vi "Config Dialog.vi"(8 "error in (no error)":errorcluster, 11 "DataGrid Config in":refnum<class "DataGrid Config.lvclass">) -> (0 "error out":errorcluster, 3 "DataGrid Config out":refnum<class "DataGrid Config.lvclass">)   [LabVIEW 2018, in "DataGrid Config Dialog.lvclass"]
uses:
  DataGrid Config Dialog.lvclass
  DataGrid Config/DataGrid Config.lvclass
  DataGrid Config Dialog.lvclass/DataGrid Config Dialog.ctl
panel:
  in  "Down":bool
  in  "Up":bool
  in  "Remove":bool
  in  "Add":bool
  in  "Selection":i32(listbox)
  in  "OK":bool
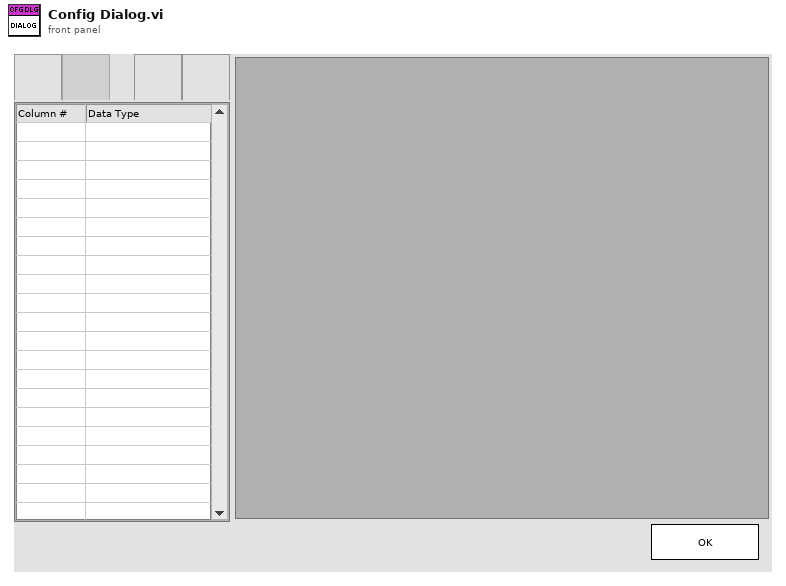
[diagram p1: front panel]
types:
  T1 = typedef "LVPoint32TypeDef.ctl" = cluster{"Horizontal":i32, "Vertical":i32}
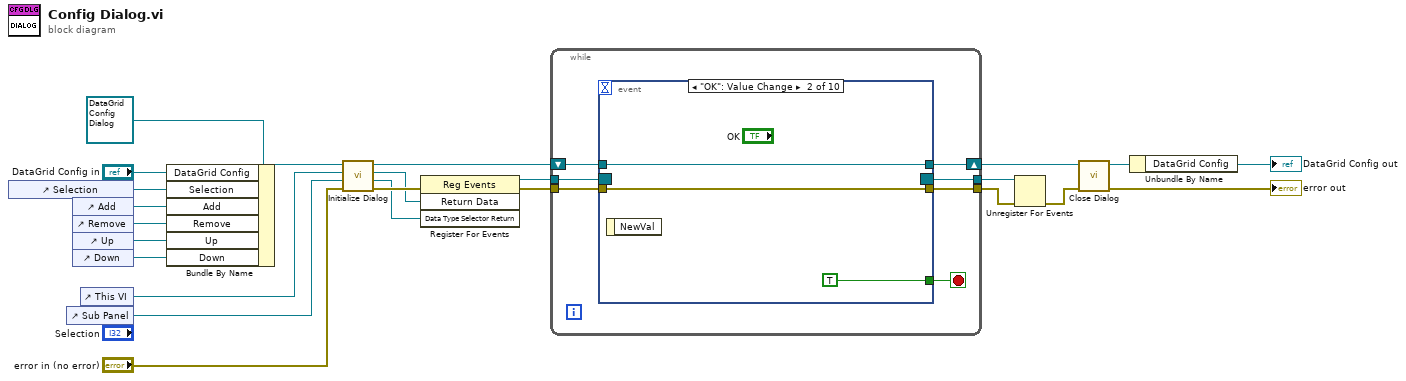
[diagram p0: block diagram]
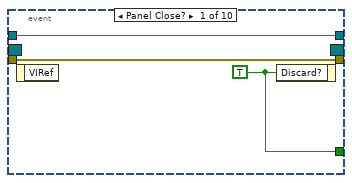
[diagram p2: hidden frame]
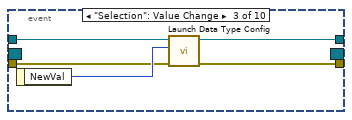
[diagram p3: hidden frame]
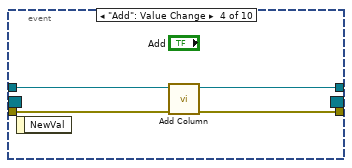
[diagram p4: hidden frame]
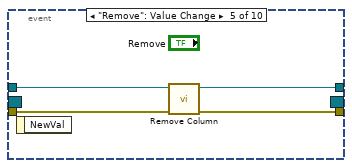
[diagram p5: hidden frame]
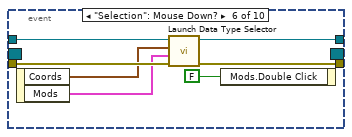
[diagram p6: hidden frame]
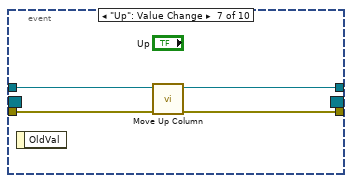
[diagram p7: hidden frame]
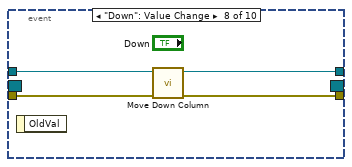
[diagram p8: hidden frame]
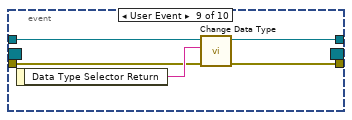
[diagram p9: hidden frame]
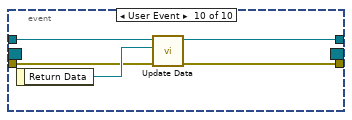
[diagram p10: hidden frame]
diagram:
  n1 = control-ref of="Selection"() -> (w22:refnum<vi>)
  n2 = control-ref of="Sub Panel"() -> (w21:refnum<vi>)
  n3 = control-ref of="Add"() -> (w11:refnum<vi>)
  n4 = control-ref of="Remove"() -> (w10:refnum<vi>)
  n5 = control-ref of="Up"() -> (w7:refnum<vi>)
  n6 = control-ref of="Down"() -> (w6:refnum<vi>)
  n7 = control-ref of="This VI"() -> (w20:refnum<vi>)
  n8 = Bundle By Name(cluster=refnum<class "DataGrid Config Dialog.lvclass"> refnum ("DataGrid Config Dialog.lvclass"), "DataGrid Config"="DataGrid Config in", "Selection"=w22, "Add"=w11, "Remove"=w10, "Up"=w7, "Down"=w6) -> (w4:refnum<class "DataGrid Config Dialog.lvclass">)
  n9 = call "Initialize Dialog.vi"("error in (no error)"="error in (no error)", "SubPnl Refnum"=w21, "VI Refnum"=w20, "DataGrid Config Dialog in"=w4) -> ("error out"=w23:errorcluster, "Data Type Selector Return"=w8:refnum<user-event>, "Return Data"=w15:refnum<user-event>, "DataGrid Config Dialog out"=w24:refnum<class "DataGrid Config Dialog.lvclass">)  [unwired: 4 in]
  n10 = register-events(error in=w23, w15, w8) -> (reference out=w14:refnum<event-registration>, error out=w16:errorcluster)  [unwired: 1 in]
  n11 = while {
    shift-right: [w31] -> w19
    shift-left: w24 -> [w30]
    tunnel: w16 -> [w28]
    tunnel: w14 -> [w27]
    tunnel: [w26] -> w13
    tunnel: [w25] -> w1
    stop <- w29 stop-if-true
    n12 = event shown="[1] \"OK\": Value Change" {
      selector: w27 -> [_ _ _ _ _ _ _ _ _ _]
      dyn-events: [_ _ _ _ _ _ _ _ _ _] -> w26
      timeout: _ -> [_ _ _ _ _ _ _ _ _ _]
      tunnel: [w34 w37 w41 w45 w48 w52 w59 w63 w67 w74] -> w31
      tunnel: w30 -> [w34 w37 w42 w46 w50 w56 w61 w65 w70 w75]
      tunnel: [w33 TRUE ("Discard?") _ _ _ _ _ _ _ _] -> w29
      tunnel: w28 -> [w32 w35 w39 w44 w49 w55 w60 w64 w68 w72]
      tunnel: [w32 w35 w38 w43 w47 w51 w58 w62 w66 w71] -> w25
      event Panel Close? {
        w33 = TRUE ("Discard?")
        n13 = event-data() -> ()  [unwired: 1 in, 1 out]
        n14 = event-data("Discard?"=w33) -> ()  [unwired: 1 in, 1 out]
      }
      event "OK": Value Change {
        n15 = event-data() -> ()  [unwired: 1 in, 1 out]
      }
      event "Selection": Value Change {
        n16 = event-data() -> ("NewVal"=w40:i32)  [unwired: 1 in]
        n17 = call "Launch Data Type Config.vi"("error in (no error)"=w39, "Selection"=w40, "DataGrid Config Dialog in"=w42) -> ("error out"=w38:errorcluster, "DataGrid Config Dialog out"=w41:refnum<class "DataGrid Config Dialog.lvclass">)  [unwired: 7 in]
      }
      event "Add": Value Change {
        n18 = event-data() -> ()  [unwired: 1 in, 1 out]
        n19 = call "Add Column.vi"("error in (no error)"=w44, "DataGrid Config Dialog in"=w46) -> ("error out"=w43:errorcluster, "DataGrid Config Dialog out"=w45:refnum<class "DataGrid Config Dialog.lvclass">)  [unwired: 8 in]
      }
      event "Remove": Value Change {
        n20 = event-data() -> ()  [unwired: 1 in, 1 out]
        n21 = call "Remove Column.vi"("error in (no error)"=w49, "DataGrid Config Dialog in"=w50) -> ("error out"=w47:errorcluster, "DataGrid Config Dialog out"=w48:refnum<class "DataGrid Config Dialog.lvclass">)  [unwired: 8 in]
      }
      event "Selection": Mouse Down? {
        n22 = event-data() -> ("Coords"=w54:T1, "Mods"=w53:cluster{"Double Click":bool, "Menu Key":bool})  [unwired: 1 in]
        n23 = call "Launch Data Type Selector.vi"("error in (no error)"=w55, "Mods"=w53, "Coords"=w54, "DataGrid Config Dialog in"=w56) -> ("error out"=w51:errorcluster, "DataGrid Config Dialog out"=w52:refnum<class "DataGrid Config Dialog.lvclass">)  [unwired: 6 in]
        n24 = event-data("Mods.Double Click"=FALSE ("Double Click")) -> ()  [unwired: 1 in, 1 out]
      }
      event "Up": Value Change {
        n25 = event-data() -> ()  [unwired: 1 in, 1 out]
        n26 = call "Move Up Column.vi"("error in (no error)"=w60, "DataGrid Config Dialog in"=w61) -> ("error out"=w58:errorcluster, "DataGrid Config Dialog out"=w59:refnum<class "DataGrid Config Dialog.lvclass">)  [unwired: 8 in]
      }
      event "Down": Value Change {
        n27 = event-data() -> ()  [unwired: 1 in, 1 out]
        n28 = call "Move Down Column.vi"("error in (no error)"=w64, "DataGrid Config Dialog in"=w65) -> ("error out"=w62:errorcluster, "DataGrid Config Dialog out"=w63:refnum<class "DataGrid Config Dialog.lvclass">)  [unwired: 8 in]
      }
      event User Event {
        n29 = event-data() -> ("Data Type Selector Return"=w69:string)  [unwired: 1 in]
        n30 = call "Change Data Type.vi"("error in (no error)"=w68, "Data Type Selector Return"=w69, "DataGrid Config Dialog in"=w70) -> ("error out"=w66:errorcluster, "DataGrid Config Dialog out"=w67:refnum<class "DataGrid Config Dialog.lvclass">)  [unwired: 7 in]
      }
      event User Event {
        n31 = event-data() -> ("Return Data"=w73:refnum<class "Generic Data Type.lvclass">)  [unwired: 1 in]
        n32 = call "Update Data.vi"("error in (no error)"=w72, "Generic Data Type"=w73, "DataGrid Config Dialog in"=w75) -> ("error out"=w71:errorcluster, "DataGrid Config Dialog out"=w74:refnum<class "DataGrid Config Dialog.lvclass">)  [unwired: 7 in]
      }
    }
  }
  n33 = Unregister For Events(event registration refnum=w13, error in=w1) -> (error out=w12:errorcluster)
  n34 = call "Close Dialog.vi"("error in (no error)"=w12, "DataGrid Config Dialog in"=w19) -> ("error out"=→"error out":errorcluster, "DataGrid Config Dialog out"=w18:refnum<class "DataGrid Config Dialog.lvclass">)  [unwired: 8 in]
  n35 = Unbundle By Name(w18) -> ("DataGrid Config"=→"DataGrid Config out":refnum<class "DataGrid Config.lvclass">)
